vi "build raw waveform.vi"(11 "Y":dbl[](array[numeric])) -> (3 "Raw Waveform Data":u8[](array[numeric]) format="%x")   [LabVIEW 2021]
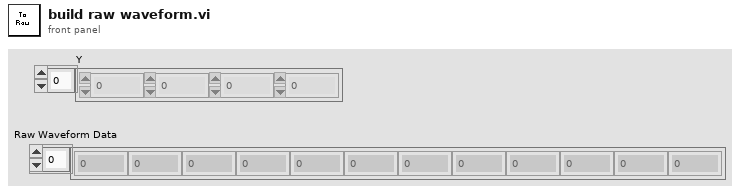
[diagram p1: front panel]
types:
  T1 = enum16{"big-endian, network order", "native, host order", "little-endian"}
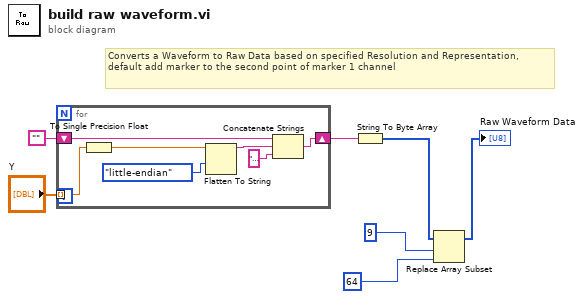
[diagram p0: block diagram]
diagram:
  # "Converts a Waveform to Raw Data based on specified Resolution and Representation, default add marker to the second point of marker 1 channel"
  n1 = for {
    tunnel: "Y" -> [w14] mode=indexing
    shift-right: [w8] -> w6
    shift-left: "" ("Empty String Constant") -> [w11]
    n2 = To Single Precision Float(number=w14) -> (single precision float=w13:sgl)
    n3 = Flatten To String(anything=w13, byte order (0:big-endian, network order)=T1."little-endian") -> (data string=w10:string)  [unwired: 2 in, 2 out]
    n4 = Concatenate Strings(w11, w10, "\u0000" ("string")) -> (w8:string)
  }
  n5 = String To Byte Array(string=w6) -> (unsigned byte array=w4:u8[])
  n6 = Replace Array Subset(array=w4, new element=u8 64 ("new element/subarray"), index=9) -> (→"Raw Waveform Data":u8[])
